vi "LDA mirror adjust.vi"(1 "Mirror Up?":bool) -> (0 "Error String":string)   [LabVIEW 2022 SP3]
uses:
  Anemometry/Anemometry Sub Vis/Globals/Constants_global.vi
  Anemometry/Anemometry Sub Vis/Globals/Trav_pos_global.vi
panel:
  in  "Drive mirror up and down again":bool
  out "write buffer":string="p2198\r"
  out "UP posn":i16=809 min=750 max=2250
  out "DOWN posn":i16=2198 min=750 max=2250
  # "750 MIN\n\n\n\n2250 MAX"
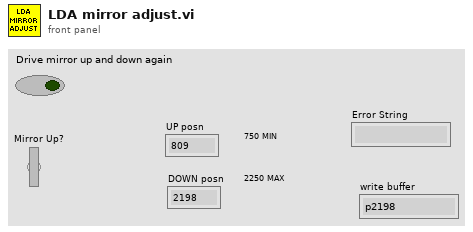
[diagram p1: front panel]
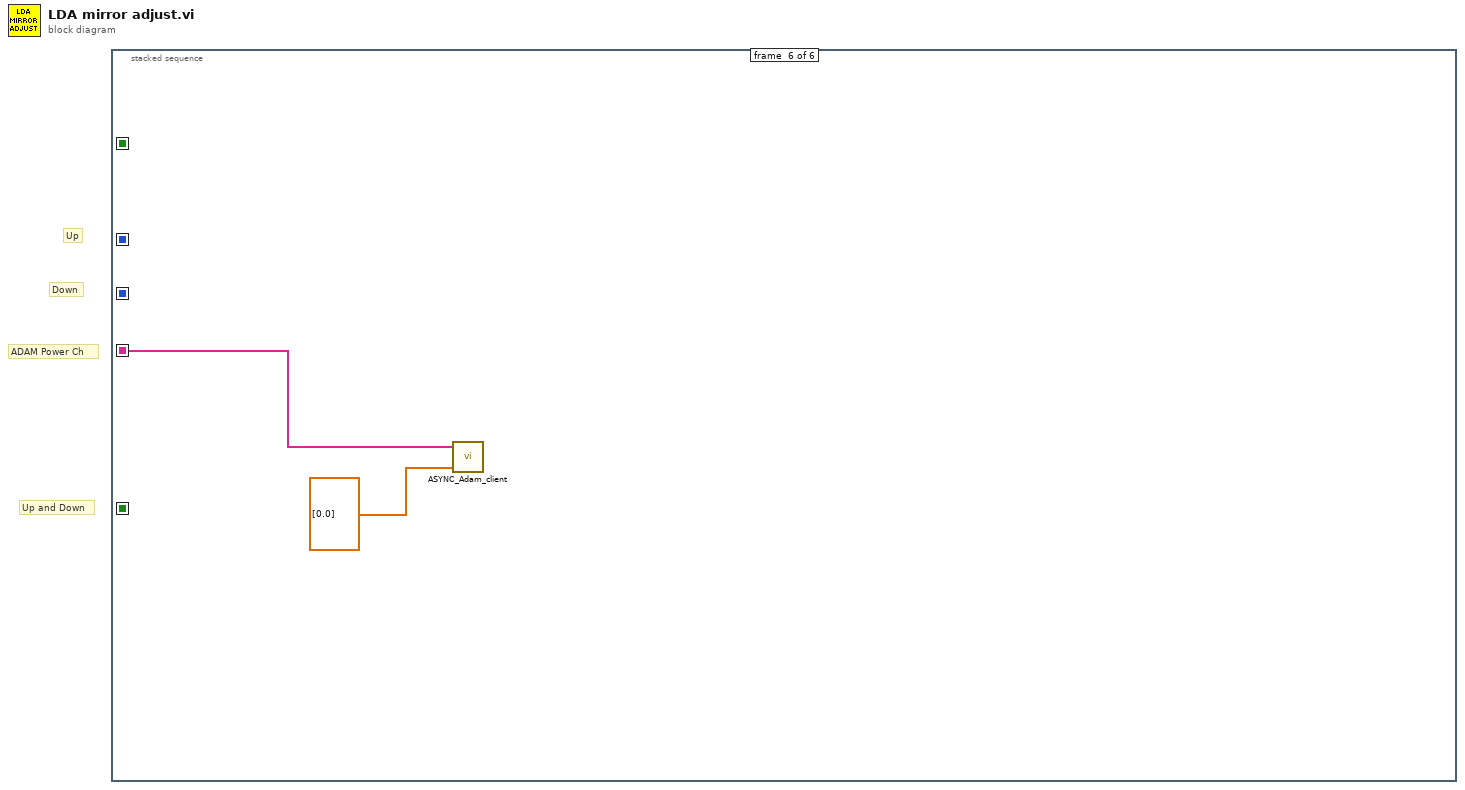
[diagram p0: block diagram]
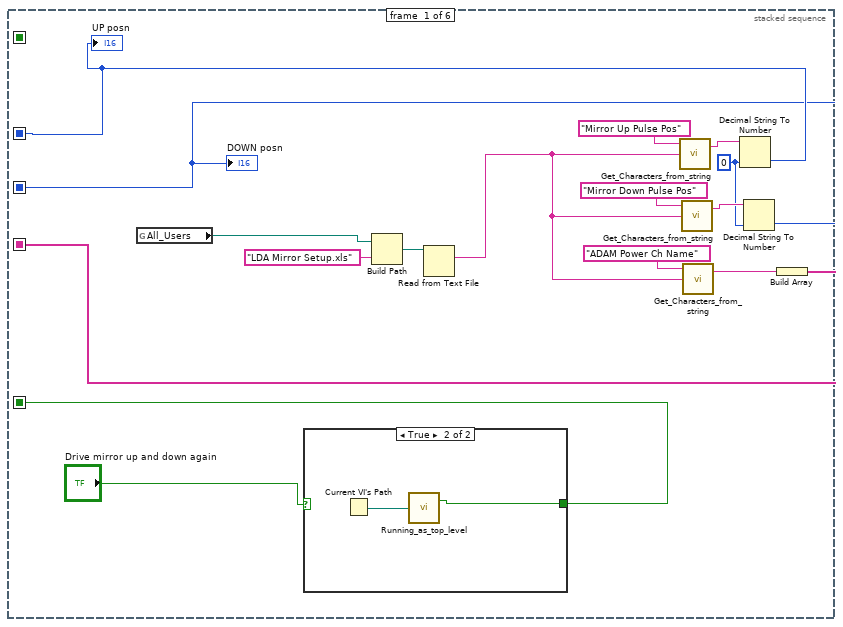
[diagram p2: hidden frame]
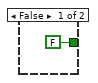
[diagram p3: hidden frame]
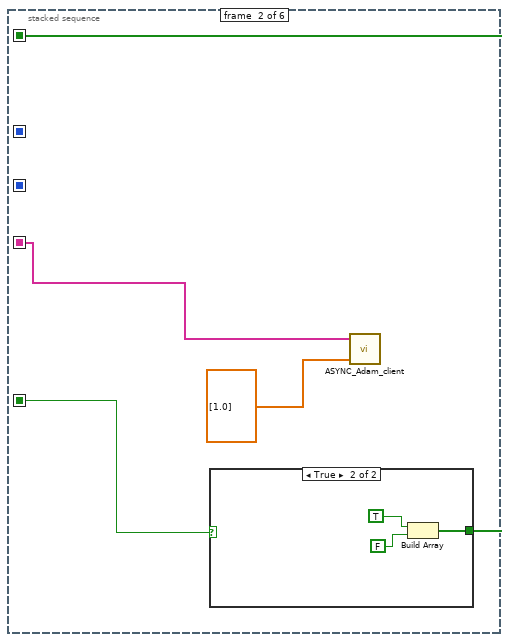
[diagram p4: hidden frame]
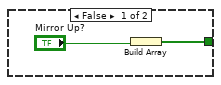
[diagram p5: hidden frame]
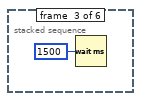
[diagram p6: hidden frame]
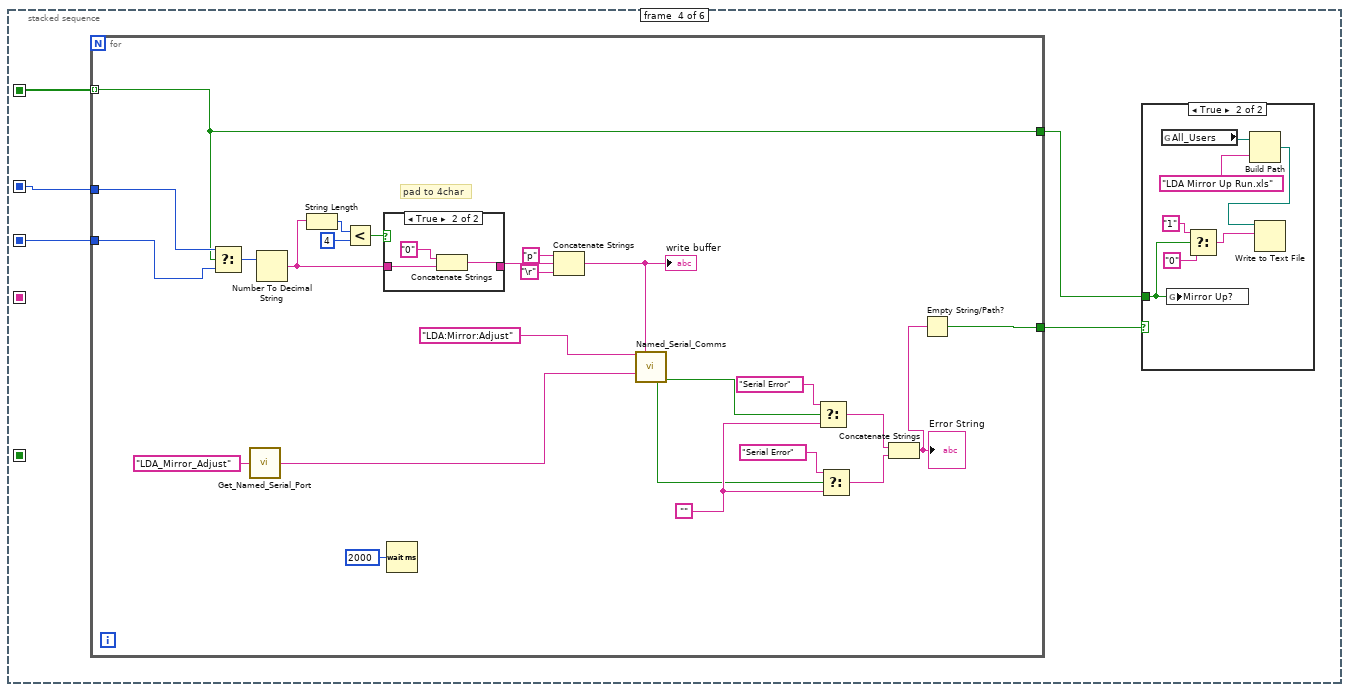
[diagram p7: hidden frame]
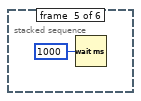
[diagram p10: hidden frame]
diagram:
  # "Up and Down"
  # "ADAM Power Ch"
  # "Down"
  # "Up"
  n1 = stacked-sequence {
    seq-local: [w2 _ _ _ _ _] -> [_ _ _ w33 _ _]
    seq-local: [w1 _ _ _ _ _] -> [_ _ _ w32 _ _]
    seq-local: [w5 _ _ _ _ _] -> [_ w23 _ _ _ w72]
    seq-local: [w3 _ _ _ _ _] -> [_ w20 _ _ _ _]
    seq-local: [_ w21 _ _ _ _] -> [_ _ _ w31 _ _]
    frame #0 {
      w8 = i16 0 ("default (0 I32)")
      n2 = global read "Constants_global.vi" "All_Users"() -> (w13:path)
      n3 = case shown="True" "Drive mirror up and down again" {
        tunnel: [FALSE ("Top Level") w18] -> w3
        frame False {
        }
        frame True {
          n4 = Current VI's Path() -> (path=w19:path)
          n5 = call "Running_as_top_level.vi"("Vi path name"=w19) -> ("Top Level"=w18:bool)  [unwired: 1 out]
        }
      }
      n6 = Build Path(base path=w13, name or relative path="LDA Mirror Setup.xls") -> (appended path=w14:path)
      n7 = Read from Text File(file (use dialog)=w14) -> (text=w7:string)  [unwired: 3 in, 3 out]
      n8 = call "Get_Characters_from_string.vi"("Input string"=w7, "Variable name"="Mirror Up Pulse Pos") -> ("Value"=w10:string)  [unwired: 1 in, 1 out]
      n9 = call "Get_Characters_from_string.vi"("Input string"=w7, "Variable name"="Mirror Down Pulse Pos") -> ("Value"=w9:string)  [unwired: 1 in, 1 out]
      n10 = call "Get_Characters_from_string.vi"("Input string"=w7, "Variable name"="ADAM Power Ch Name") -> ("Value"=w6:string)  [unwired: 1 in, 1 out]
      n11 = Decimal String To Number(string=w10, default (0L)=w8) -> (number=w2:i16)  [unwired: 1 in, 1 out]
      "UP posn" <- w2
      n12 = Decimal String To Number(string=w9, default (0L)=w8) -> (number=w1:i16)  [unwired: 1 in, 1 out]
      "DOWN posn" <- w1
      n13 = Build Array(w6) -> (w5:string[])
    }
    frame #1 {
      n14 = case shown="True" w20 {
        tunnel: [w24 w26] -> w21
        frame False {
          n15 = Build Array("Mirror Up?") -> (w24:bool[])
        }
        frame True {
          n16 = Build Array(TRUE ("Mirror Up?"), FALSE ("Mirror Up?")) -> (w26:bool[])
        }
      }
      n17 = call "ASYNC_Adam_client.vi"("Values"=dbl[] [1.0], "Channel Names"=w23) -> ()  [unwired: 1 in, 2 out]
    }
    frame #2 {
      n18 = Wait (ms)(milliseconds to wait=u32 1500) -> ()  [unwired: 1 out]
    }
    frame #3 {
      n19 = for {
        tunnel: [w41] -> w34
        tunnel: w33 -> [w38]
        tunnel: w32 -> [w37]
        tunnel: w31 -> [w36] mode=indexing
        tunnel: [w36] -> w30
        w46 = ""
        # "pad to 4char"
        n20 = Select(t=w38, s=w36, f=w37) -> (s? t:f=w57:i16)
        n21 = call "Get_Named_Serial_Port.vi"("Serial Port Alias"="LDA_Mirror_Adjust") -> ("Serial Port Name"=w39:string)
        n22 = Number To Decimal String(number=w57) -> (decimal integer string=w53:string)  [unwired: 1 in]
        n23 = String Length(string=w53) -> (length=w56:i32)
        n24 = Less?(x=w56, y=4) -> (x < y?=w54:bool)
        n25 = case shown="True" w54 {
          tunnel: [w60 w62] -> w52
          tunnel: w53 -> [w60 w61]
          frame False {
          }
          frame True {
            n26 = Concatenate Strings("0", w61) -> (w62:string)
          }
        }
        n27 = Wait (ms)(milliseconds to wait=u32 2000) -> ()  [unwired: 1 out]
        n28 = Concatenate Strings("p", w52, "\r") -> (w51:string)
        "write buffer" <- w51
        n29 = call "Named_Serial_Comms.vi"("Channel Name"="LDA:Mirror:Adjust" ("Ch Name"), "Write"=w51, "Port Name"=w39) -> ("Timed out"=w45:bool, "Serial Error"=w49:bool)  [unwired: 6 in, 5 out]
        n30 = Select(t="Serial Error", s=w49, f=w46) -> (s? t:f=w44:string)
        n31 = Select(t="Serial Error", s=w45, f=w46) -> (s? t:f=w43:string)
        n32 = Concatenate Strings(w44, w43) -> (w42:string)
        "Error String" <- w42
        n33 = Empty String/Path?(string/path=w42) -> (empty?=w41:bool)
      }
      n34 = case shown="True" w34 {
        tunnel: w30 -> [_ w66]
        frame False {
        }
        frame True {
          n35 = global read "Constants_global.vi" "All_Users"() -> (w70:path)
          n36 = global write "Trav_pos_global.vi" "Mirror Up?"(w66) -> ()
          n37 = Select(t="1" ("String to match"), s=w66, f="0" ("String to match")) -> (s? t:f=w65:string)
          n38 = Build Path(base path=w70, name or relative path="LDA Mirror Up Run.xls") -> (appended path=w64:path)
          n39 = Write to Text File(file (use dialog)=w64, text=w65) -> ()  [unwired: 2 in, 3 out]
        }
      }
    }
    frame #4 {
      n40 = Wait (ms)(milliseconds to wait=u32 1000) -> ()  [unwired: 1 out]
    }
    frame #5 {
      n41 = call "ASYNC_Adam_client.vi"("Values"=dbl[] [0.0], "Channel Names"=w72) -> ()  [unwired: 1 in, 2 out]
    }
  }
